vi "Clear Dictionary.vi"(8 "error in (no error)":errorcluster, 11 "SMO.Dictionary.Variant in":refnum<class "SMO.Dictionary.Variant.lvclass">) -> (0 "error out":errorcluster, 3 "SMO.Dictionary.Variant out":refnum<class "SMO.Dictionary.Variant.lvclass">)   [LabVIEW 2013, in "SMO.Dictionary.lvlib" / "SMO.Dictionary.Variant.lvclass"]
uses:
  SMO.Dictionary.Variant.lvclass
  SMO.Dictionary.Variant.lvclass/SMO.Dictionary.Variant.ctl
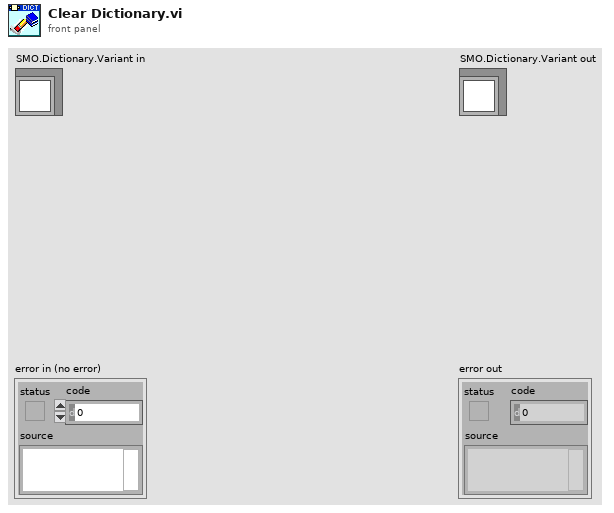
[diagram p1: front panel]
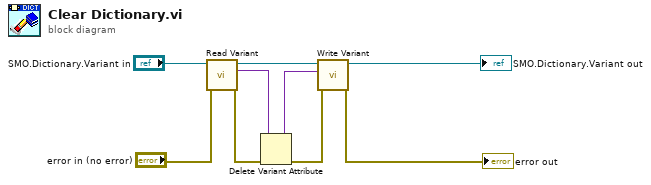
[diagram p0: block diagram]
diagram:
  n1 = call "Read Variant.vi"("error in (no error)"="error in (no error)", "SMO.Dictionary.Variant in"="SMO.Dictionary.Variant in") -> ("error out"=w3:errorcluster, "Variant"=w5:variant, "SMO.Dictionary.Variant out"=w8:refnum<class "SMO.Dictionary.Variant.lvclass">)  [unwired: 7 in]
  n2 = Delete Variant Attribute(4:w3, 7:w5) -> (0:w2:errorcluster, 3:w7:variant)  [unwired: 1 in, 1 out]
  n3 = call "Write Variant.vi"("error in (no error)"=w2, "Variant"=w7, "SMO.Dictionary.Variant in"=w8) -> ("error out"=→"error out":errorcluster, "SMO.Dictionary.Variant out"=→"SMO.Dictionary.Variant out":refnum<class "SMO.Dictionary.Variant.lvclass">)  [unwired: 7 in]
